vi "write--all.vi"(0 "DVR value":T1) -> ()   [LabVIEW 2018, in "main.lvlib" / "app_data.lvlib"]
uses:
  app_data.lvlib
  app_data.ctl
  core/core_data/core_data.ctl
  core/core_data/completed_tour.ctl
  core/core_data/chessboard_index.ctl
  core/core_data/tour_in_progress.ctl
  core/core_data/chess_square.ctl
  core/core_data/neighbour_square.ctl
  library_variable.vi
  core/core_data/core_data.lvlib
panel:
  # "Development\ncontrols/indicators useful for development and testing, but which are not outputs of the VI"
  # "Input\nInputs to the VI"
  # "Output\nOutputs of the VI"
  # "Description\n\nBlank VI with error handling case. \n\nSummarize the use of this VI in this space."
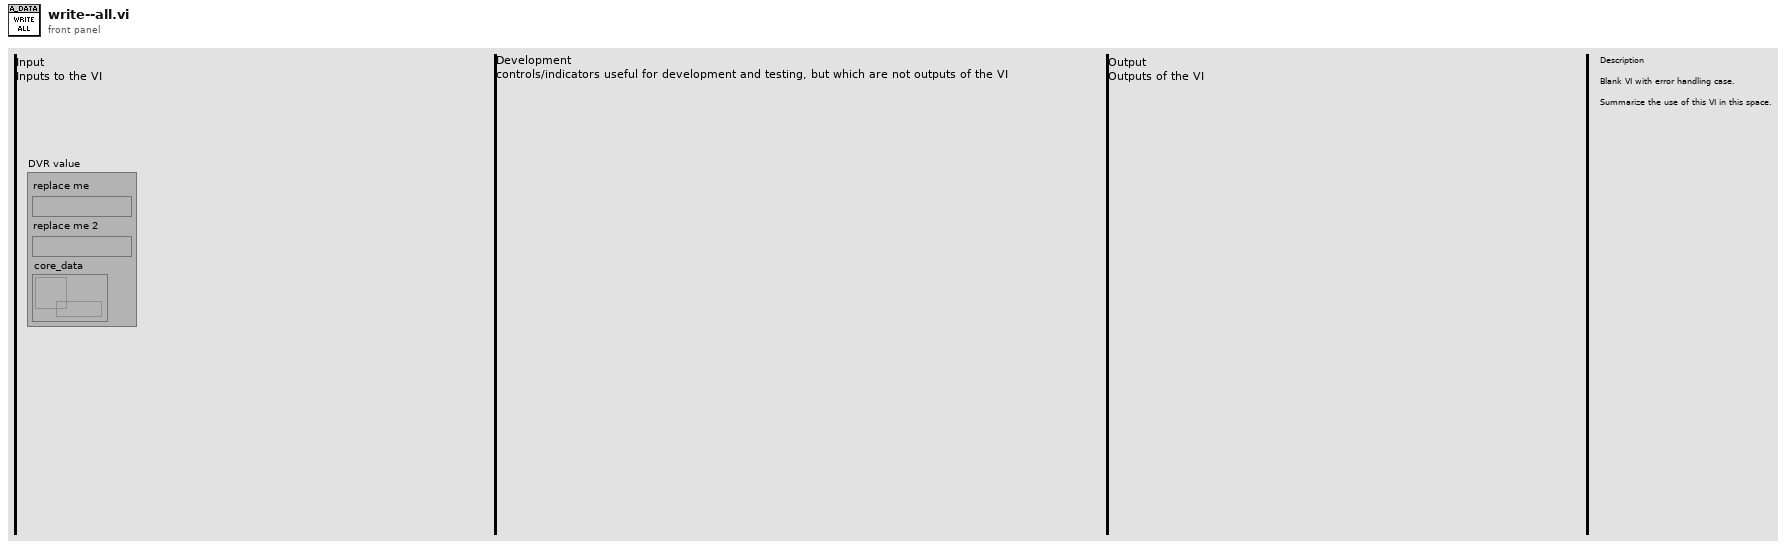
[diagram p1: front panel]
types:
  T1 = typedef "main.lvlib/app_data.lvlib/app_data.ctl" = cluster{"replace me":string, "replace me 2":string, "core_data":refnum<data-value>}
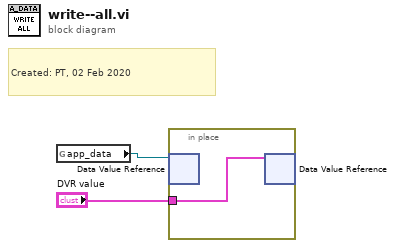
[diagram p0: block diagram]
diagram:
  # "Created: PT, 02 Feb 2020"
  n1 = global read "library_variable.vi" "app_data"() -> (w1:refnum<data-value>)
  n2 = in-place {
    in-place-border: "DVR value" -> [w3]
    n3 = in-place-dvr #1(w1) -> ()  [unwired: 2 out]
    n4 = in-place-dvr #1(w3) -> ()  [unwired: 2 out]
  }
